vi "MessageCycleCore.vi"   [LabVIEW 2019]
panel:
  # "通讯循环,用于通讯"
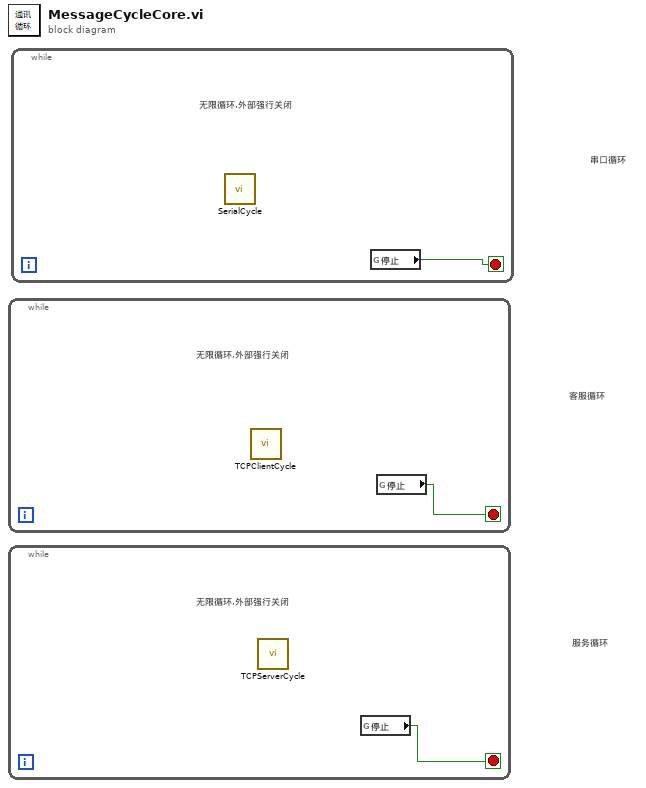
[diagram p0: block diagram]
diagram:
  # "服务循环"
  # "客服循环"
  # "串口循环"
  n1 = while {
    stop <- w1 stop-if-true
    # "无限循环,外部强行关闭"
    n2 = call "TCPClientCycle.vi"() -> ()  [unwired: 20 in]
    n3 = global read "全局-配置识别.vi" "停止"() -> (w1:bool)
  }
  n4 = while {
    stop <- w2 stop-if-true
    # "无限循环,外部强行关闭"
    n5 = call "TCPServerCycle.vi"() -> ()  [unwired: 20 in]
    n6 = global read "全局-配置识别.vi" "停止"() -> (w2:bool)
  }
  n7 = while {
    stop <- w3 stop-if-true
    # "无限循环,外部强行关闭"
    n8 = call "SerialCycle.vi"() -> ()  [unwired: 20 in]
    n9 = global read "全局-配置识别.vi" "停止"() -> (w3:bool)
  }
